vi "Measurement Logic.vi"() -> ()   [LabVIEW 2024, in "NIFgenSignalVoltageGeneration.lvlib"]
uses:
  NIFgenSignalVoltageGeneration.lvlib
  Measurement Configuration.ctl
  Measurement Results.ctl
  <vilib>/MeasurementLink/MeasurementLink Measurement Server/Measure Call Context/Measure Call Context.lvclass
  <instrlib>/niFgen/niFgen.llb/niFgen Output Mode.ctl
  <vilib>/MeasurementLink/MeasurementLink niFGEN/Initialize Sessions - 1Sess.vi
  <vilib>/MeasurementLink/MeasurementLink niFGEN/MeasurementLink niFGEN.lvlib
  <vilib>/MeasurementLink/MeasurementLink Session Management V1/Session Reservation/Session Reservation.lvclass
panel:
  out "actual duration":dbl
  out "measure call context out":refnum<class "Measure Call Context.lvclass">
  in  "measure call context in":refnum<class "Measure Call Context.lvclass">
  out "measurement results":T1
  in  "measurement configuration":T2 {"Waveform Type" items=["Sine", "Square"]}
  out "error out":errorcluster
  in  "error in":errorcluster
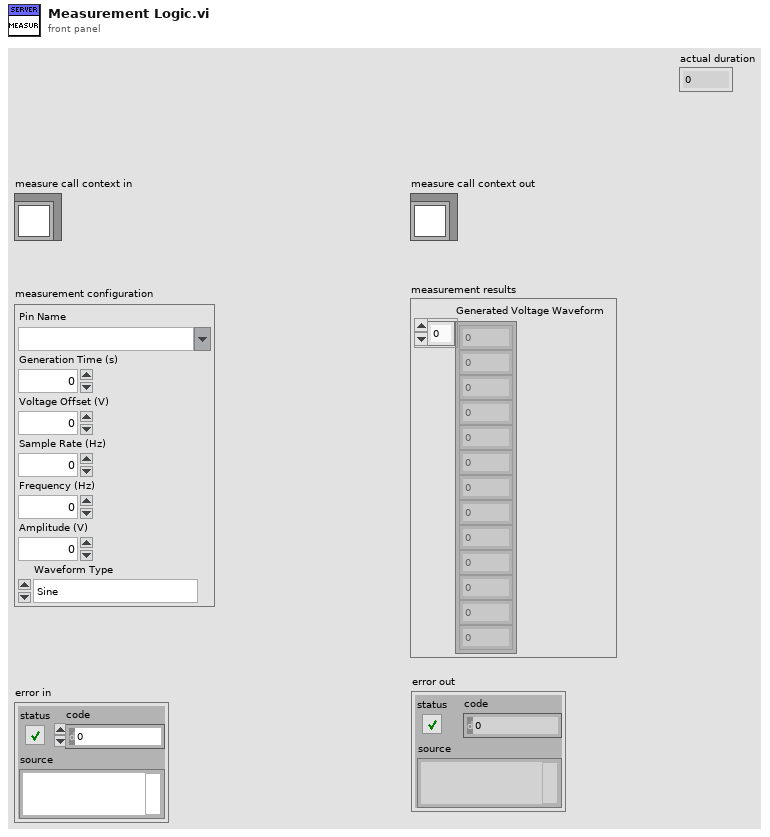
[diagram p1: front panel]
types:
  T1 = typedef "NIFgenSignalVoltageGeneration.lvlib/Measurement Results.ctl" = cluster{"Generated Voltage Waveform":dbl[]}
  T2 = typedef "NIFgenSignalVoltageGeneration.lvlib/Measurement Configuration.ctl" = cluster{"Pin Name":string, "Generation Time (s)":dbl, "Voltage Offset (V)":dbl, "Sample Rate (Hz)":dbl, "Frequency (Hz)":dbl, "Amplitude (V)":dbl, "Waveform Type":i32}
  T3 = typedef "niFgen Output Mode.ctl" = u32
  T4 = cluster{"Waveform Type":i32, "Amplitude (V)":dbl, dbl}
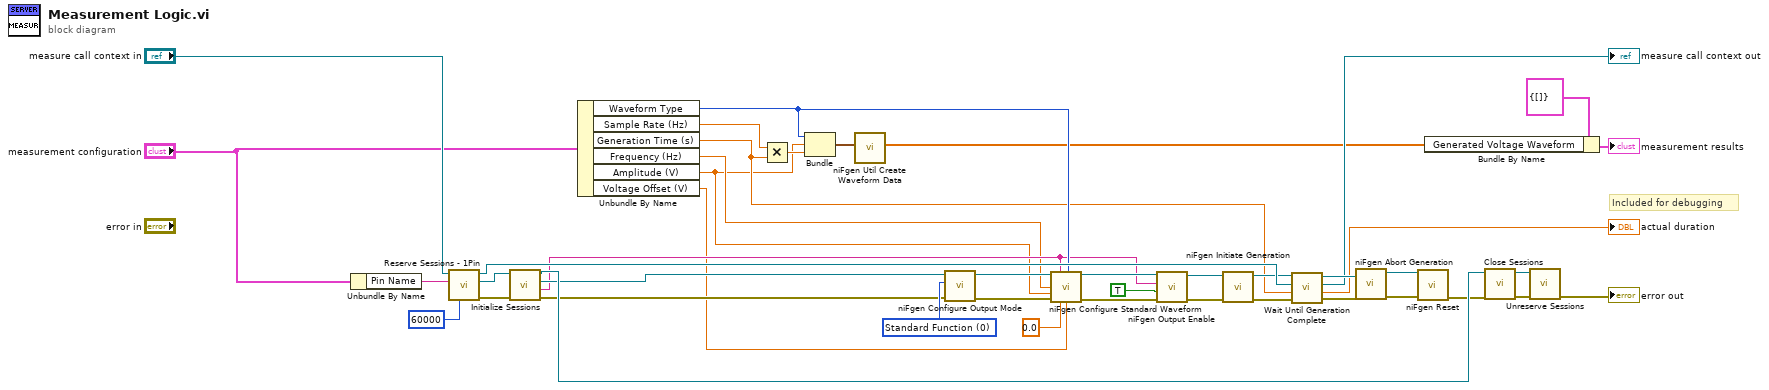
[diagram p0: block diagram]
diagram:
  w37 = T3 0 items=["Standard Function", "Frequency List", "Arbitrary Waveform", "Arbitrary Sequence", "Script"] ("Output Mode (default: 0=Standard Function)")
  # "Included for debugging"
  n1 = Unbundle By Name("measurement configuration") -> ("Pin Name"=w38:string)
  n2 = call <vilib>:"Reserve Sessions - 1Pin.vi"("timeout (ms)"=60000, "pin or relay name"=w38, "measurement context in"="measure call context in") -> ("error out"=w41:errorcluster, "session reservation out"=w40:refnum<class "Session Reservation.lvclass">, "measurement context out"=w26:refnum<class "Measure Call Context.lvclass">)  [unwired: 6 in]
  n3 = call-poly <vilib>:"Initialize Sessions.vi"("error in"=w41, "session reservation in"=w40) -> ("error out"=w28:errorcluster, "channel list"=w7:string, "session"=w27:refnum<k15>, "session reservation out"=w30:refnum<class "Session Reservation.lvclass">)  [unwired: 6 in]
  n4 = Unbundle By Name("measurement configuration") -> ("Waveform Type"=w15:i32, "Sample Rate (Hz)"=w5:dbl, "Generation Time (s)"=w6:dbl, "Frequency (Hz)"=w3:dbl, "Amplitude (V)"=w2:dbl, "Voltage Offset (V)"=w4:dbl)
  n5 = Multiply(x=w5, y=w6) -> (x*y=w14:dbl)
  n6 = Bundle("Waveform Type"=w15, "Amplitude (V)"=w2, w14) -> (w1:T4)  [unwired: 1 in]
  n7 = call <instrlib>:"niFgen Util Create Waveform Data.vi"("Waveform"=w1) -> ("Waveform Data"=w13:dbl[])  [unwired: 10 in]
  n8 = call <instrlib>:"niFgen Configure Output Mode.vi"("error in (no error)"=w28, "Output Mode (default: 0=Standard Function)"=w37, "Instrument Handle"=w27) -> ("error out"=w11:errorcluster, "Instrument Handle Out"=w12:refnum<k15>)  [unwired: 6 in]
  n9 = call <instrlib>:"niFgen Configure Standard Waveform.vi"("Instrument Handle"=w12, "Channel Name"=w7, "Waveform"=w15, "Frequency"=w3, "Amplitude"=w2, "error in (no error)"=w11, "Start Phase"=0.0, "DC Offset"=w4) -> ("Instrument Handle Out"=w10:refnum<k15>, "error out"=w9:errorcluster)  [unwired: 6 in]
  n10 = call <instrlib>:"niFgen Output Enable.vi"("error in (no error)"=w9, "Output Enable (default: True)"=TRUE, "Channel Name"=w7, "Instrument Handle"=w10) -> ("error out"=w21:errorcluster, "Instrument Handle Out"=w20:refnum<k15>)  [unwired: 6 in]
  n11 = call <instrlib>:"niFgen Initiate Generation.vi"("error in (no error)"=w21, "Instrument Handle"=w20) -> ("error out"=w18:errorcluster, "Instrument Handle Out"=w19:refnum<k15>)  [unwired: 8 in]
  n12 = call "Wait Until Generation Complete.vi"("error in"=w18, "duration"=w6, "measurement context in"=w26, "instrument handle in"=w19) -> ("error out"=w32:errorcluster, "actual duration"=→"actual duration":dbl, "measurement context out"=→"measure call context out":refnum<class "Measure Call Context.lvclass">, "instrument handle out"=w33:refnum<k15>)  [unwired: 4 in]
  n13 = call <instrlib>:"niFgen Abort Generation.vi"("error in (no error)"=w32, "Instrument Handle"=w33) -> ("error out"=w23:errorcluster, "Instrument Handle Out"=w24:refnum<k15>)  [unwired: 8 in]
  n14 = call <instrlib>:"niFgen Reset.vi"("error in (no error)"=w23, "Instrument Handle"=w24) -> ("error out"=w22:errorcluster)  [unwired: 8 in, 1 out]
  n15 = Bundle By Name(cluster=T1 {"Generated Voltage Waveform"=[]} ("Measurement Results"), "Generated Voltage Waveform"=w13) -> (→"measurement results":T1)
  n16 = call <vilib>:"Close Sessions.vi"("error in"=w22, "session reservation in"=w30) -> ("error out"=w31:errorcluster, "session reservation out"=w34:refnum<class "Session Reservation.lvclass">)  [unwired: 8 in]
  n17 = call <vilib>:"Unreserve Sessions.vi"("error in"=w31, "session reservation in"=w34) -> ("error out"=→"error out":errorcluster)  [unwired: 9 in]
